vi "Create Folder.vi"(8 "error in (no error)":errorcluster, 10 "File Name":string, 11 "Base Path":path) -> (0 "error out":errorcluster, 2 "Result File path":path, 3 "Result Folder path":path)   [LabVIEW 2022 SP3]
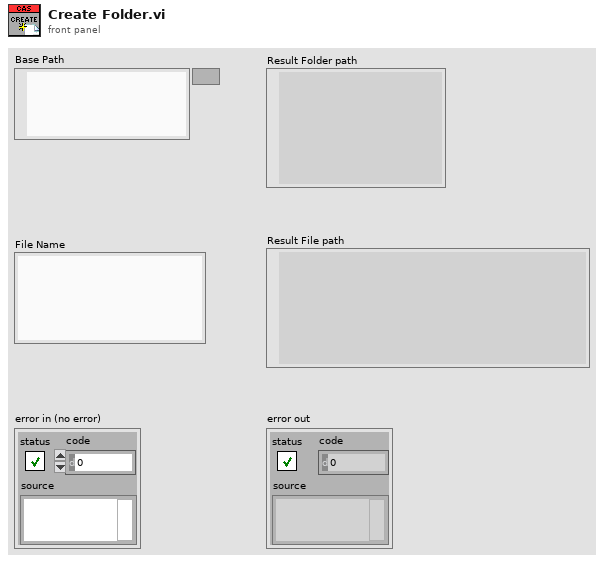
[diagram p1: front panel]
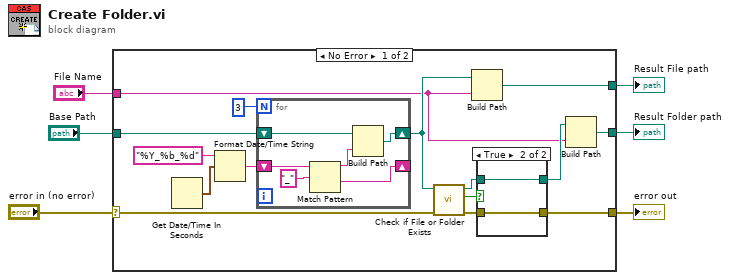
[diagram p0: block diagram]
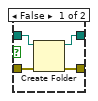
[diagram p2: hidden frame]
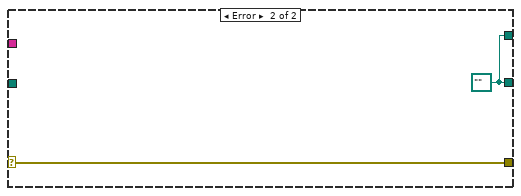
[diagram p3: hidden frame]
diagram:
  n1 = case shown="No Error" "error in (no error)" {
    selector: "error in (no error)" -> [w16 w35]
    tunnel: [w19 w35] -> w5
    tunnel: [w7 w34] -> w6
    tunnel: [w18 w34] -> w4
    tunnel: "File Name" -> [w8 _]
    tunnel: "Base Path" -> [w20 _]
    frame No Error {
      n2 = Get Date/Time In Seconds() -> (seconds since 1Jan1904=w12:timestamp)
      n3 = Format Date/Time String(time format string (%c)="%Y_%b_%d", seconds (now)=w12) -> (date/time string=w11:string)  [unwired: 1 in]
      n4 = for {
        N: 3 -> [_]
        shift-right: [w30] -> _
        shift-left: w11 -> [w28]
        shift-right: [w31] -> w9
        shift-left: w20 -> [w32]
        n5 = Match Pattern(string=w28, regular expression="_" ("search string/char (-)")) -> (before substring=w29:string, after substring=w30:string)  [unwired: 1 in, 2 out]
        n6 = Build Path(base path=w32, name or relative path=w29) -> (appended path=w31:path)
      }
      n7 = call <vilib>:"Check if File or Folder Exists.vi"("error in (no error)"=w16, "path"=w9) -> ("error out"=w14:errorcluster, "file or folder exists?"=w13:bool, "dup path"=w15:path)  [unwired: 7 in]
      n8 = Build Path(base path=w9, name or relative path=w8) -> (appended path=w7:path)
      n9 = case shown="True" w13 {
        tunnel: [w25 w26] -> w19
        tunnel: [w24 w27] -> w17
        tunnel: w15 -> [w23 w27]
        tunnel: w14 -> [w22 w26]
        frame False {
          n10 = Create Folder(path (use dialog)=w23, error in=w22) -> (created path=w24:path, error out=w25:errorcluster)  [unwired: 1 in, 1 out]
        }
        frame True {
        }
      }
      n11 = Build Path(base path=w17, name or relative path=w8) -> (appended path=w18:path)
    }
    frame Error {
      w34 = path "" ("appended path")
    }
  }
  "error out" <- w5
  "Result Folder path" <- w4
  "Result File path" <- w6
